vi "Config Setpoints.vi"(0 "reference in":refnum<class "Stand.lvclass">, 11 "error in (no error)":errorcluster) -> (15 "error out":errorcluster)   [LabVIEW 2019, in "Stand.lvclass"]
uses:
  Stand.lvclass
  D:/GIT H4000/H4000/src/Device_class/Device.lvclass
  Device_class/Device.lvclass/Device.ctl
  Stand.lvclass/Stand.ctl
  AI_class/AI.lvclass/AI.ctl
  PiecedLinearScale_class/Scale_PiecedLinear.lvclass/Scale_PiecedLinear.ctl
  <vilib>/gmath/interp.llb/Interpolate 1D.vi
  <vilib>/Utility/error.llb/Error Cluster From Error Code.vi
  FPGA_API_class/FPGA API.lvclass
  PiecedLinearScale_class/Scale_PiecedLinear.lvclass
  AI_class/AI.lvclass
  Device_class/Device.lvclass
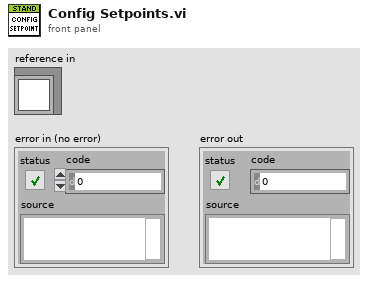
[diagram p1: front panel]
types:
  T1 = enum16{"Inlet DUT", "Outlet DUT", "StepDrive DUT", "Inlet Chamber", "Outlet Chamber", "StepDrive Chamber"}
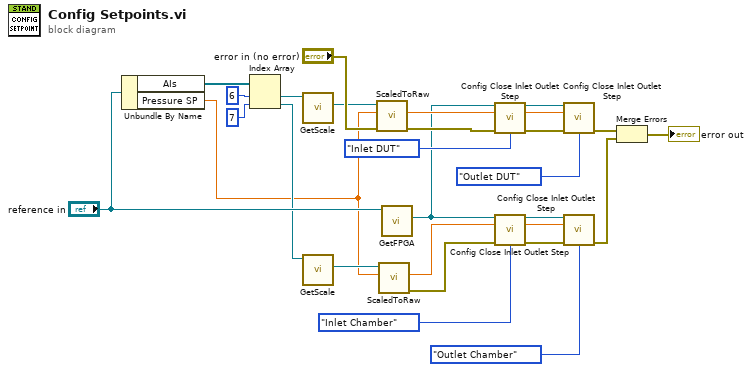
[diagram p0: block diagram]
diagram:
  n1 = Unbundle By Name("reference in") -> ("AIs"=w25:refnum<class "AI.lvclass">[], "Pressure SP"=w4:dbl)
  n2 = Index Array(array=w25, index #1=6 ("index"), index #2=7 ("index")) -> (element #1=w23:refnum<class "AI.lvclass">, element #2=w14:refnum<class "AI.lvclass">)
  n3 = call "GetScale.vi"("AI in"=w23) -> ("Scale_PiecedLinear.lvclass"=w22:refnum<class "Scale_PiecedLinear.lvclass">)  [unwired: 10 in]
  n4 = call "GetScale.vi"("AI in"=w14) -> ("Scale_PiecedLinear.lvclass"=w6:refnum<class "Scale_PiecedLinear.lvclass">)  [unwired: 10 in]
  n5 = call "ScaledToRaw.vi"("error in (no error)"="error in (no error)", "Scaled"=w4, "PiecedLinearScale in"=w22) -> ("error out"=w28:errorcluster, "Raw"=w26:dbl)  [unwired: 6 in, 1 out]
  n6 = call "ScaledToRaw.vi"("Scaled"=w4, "PiecedLinearScale in"=w6) -> ("error out"=w7:errorcluster, "Raw"=w8:dbl)  [unwired: 7 in, 1 out]
  n7 = call "GetFPGA.vi"("Device in"="reference in") -> ("FPGA API.lvclass"=w3:refnum<class "FPGA API.lvclass">)  [unwired: 10 in]
  n8 = call-dynamic "Config Close Inlet Outlet Step.vi"("FPGA API in"=w3, "sp [mA]"=w26, "error in (no error)"=w28, "Enum"=T1."Inlet DUT") -> ("FPGA API out"=w18:refnum<class "FPGA API.lvclass">, "sp [mA] dub"=w19:dbl, "error out"=w20:errorcluster)  [unwired: 9 in]
  n9 = call-dynamic "Config Close Inlet Outlet Step.vi"("FPGA API in"=w3, "sp [mA]"=w8, "error in (no error)"=w7, "Enum"=T1."Inlet Chamber") -> ("FPGA API out"=w12:refnum<class "FPGA API.lvclass">, "sp [mA] dub"=w11:dbl, "error out"=w10:errorcluster)  [unwired: 9 in]
  n10 = call-dynamic "Config Close Inlet Outlet Step.vi"("FPGA API in"=w18, "sp [mA]"=w19, "error in (no error)"=w20, "Enum"=T1."Outlet DUT") -> ("error out"=w1:errorcluster)  [unwired: 9 in, 2 out]
  n11 = call-dynamic "Config Close Inlet Outlet Step.vi"("FPGA API in"=w12, "sp [mA]"=w11, "error in (no error)"=w10, "Enum"=T1."Outlet Chamber") -> ("error out"=w5:errorcluster)  [unwired: 9 in, 2 out]
  n12 = Merge Errors(w1, w5) -> (→"error out":errorcluster)
